vi "Send subfolder levels.vi"(8 "error in (no error)":errorcluster, 11 "ImageStack in":refnum<class "ImageStack.lvclass">) -> (0 "error out":errorcluster, 3 "ImageStack out":refnum<class "ImageStack.lvclass">)   [LabVIEW 2012, in "ImageStack.lvclass"]
uses:
  ImageStack.lvclass
  ImageStack.lvclass/ImageStack.ctl
  <vilib>/Distrio/Murmex/Murmex/update_cluster.ctl
  <vilib>/Distrio/Murmex/Murmex/Murmex.lvclass
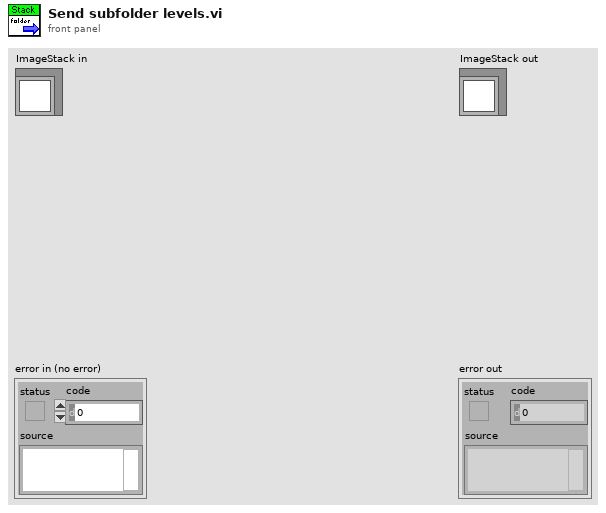
[diagram p1: front panel]
types:
  T1 = typedef "Murmex.lvlib/Murmex.lvclass/update_cluster.ctl" = cluster{"target ID":string, "key chains":string[], "values":variant[]}
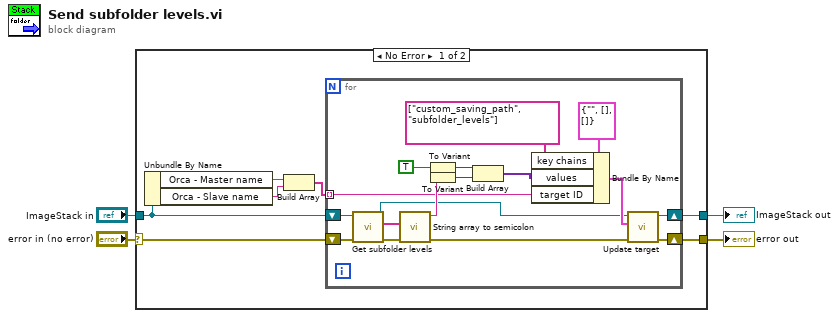
[diagram p0: block diagram]
diagram:
  n1 = case shown="No Error" "error in (no error)" {
    selector: "error in (no error)" -> [w9 w30]
    tunnel: [w11 w30] -> w3
    tunnel: [w10 w29] -> w1
    tunnel: "ImageStack in" -> [w8 w29]
    frame No Error {
      n2 = Unbundle By Name(w8) -> ("Orca - Master name"=w7:string, "Orca - Slave name"=w6:string)
      n3 = Build Array(w7, w6) -> (w5:string[])
      n4 = for {
        shift-right: [w26] -> w10
        shift-left: w8 -> [w24]
        shift-right: [w28] -> w11
        shift-left: w9 -> [w23]
        tunnel: w5 -> [w12] mode=indexing
        n5 = call-dynamic "Get subfolder levels.vi"("error in (no error)"=w23, "ImageStack in"=w24) -> ("error out"=w22:errorcluster, "Subfolder levels"=w19:string[], "ImageStack out"=w13:refnum<class "ImageStack.lvclass">)  [unwired: 7 in]
        n6 = call "String array to semicolon.vi"("error in"=w22, "String array"=w19) -> ("error out"=w14:errorcluster, "Semicolon string"=w21:string)  [unwired: 8 in]
        n7 = To Variant(anything=TRUE) -> (Variant=w15:variant)
        n8 = To Variant(anything=w21) -> (Variant=w20:variant)
        n9 = Build Array(w15, w20) -> (w17:variant[])
        n10 = Bundle By Name(cluster=T1 {"target ID"="", "key chains"=[], "values"=[]} ("update cluster"), "key chains"=string[] ["custom_saving_path", "subfolder_levels"], "values"=w17, "target ID"=w12) -> (w18:T1)
        n11 = call <vilib>:"Update target.vi"("error in (no error)"=w14, "update cluster"=w18, "MurmexBase in"=w13) -> ("error out"=w28:errorcluster, "MurmexBase out"=w26:refnum<class "ImageStack.lvclass">)  [unwired: 7 in]
      }
    }
    frame Error {
    }
  }
  "error out" <- w3
  "ImageStack out" <- w1
